vi "New Main.vi"() -> ()   [LabVIEW 2020]
panel:
  in  "Charging Voltage":dbl
  out "Total\nTemperature Change":dbl=nan
  out "Energy Loss":dbl=nan
  out "Power Loss":dbl=nan
  out "Charging Time":dbl=nan
  in  "Charing Current":dbl
  in  "Plot If Lit Up, Calculate Single if Not":bool=TRUE
  out "Results":cluster{"Output Array":dbl[], "Array y":dbl[]}(graph)
  in  "Upper Bound":dbl=2500.0
  in  "Number of Steps":dbl=2500.0
  in  "Lower Bound":dbl
  in  "Dependent Variable":u16(ring)=11 items=["Cap: Capacitance of 1 Pair NS", "Cap: Energy", "Cap: 1 NS Pair Energy / Mass", "Cap: 1 NS Pair Energy / Volume", "Cap: Impedance", "Cap: Power", "Cap: Chip Energy / Mass", "Cap: Chip Energy / Volume", "Cap: Chip Capacitance", "Cap: Chip Energy", "Cap: Chip Energy Wh", "Cap: Wh / kg", "Cap: Wh / m3", "Cap: Chip Impedance", "Cap: Chip Power", "Cap: Wh / Lit", "Cap: Energy Density Wh / m3", "Cap: J in 1 NS Pair with Gap", "Cap: Energy (Wh / m3) / 1 NS Pair with Gap", "Functionalization Molecule: Volume of Molecule", "Functionalization Molecule: Area of Molecule on CNT Surface", "Functionalization Molecule: Molecule Area with Gap", "Functionalization Molecule: Molecule Length", "Analyte Attached to Functionalized NS: Capacitance Functional Analyte per Unit Area", "Analyte Attached to Functionalized NS: Capacitance per CNT Analyte", "Analyte Attached to Functionalized NS: Capacitance Functional Analyte per NS", "Analyte Attached to Functionalized NS: Capacitance Functional Analyte per NS 2", "Analyte Molecule: Volume of Molecule Analyte", "Analyte Molecule: Area of Molecule on CNT Surface Analyte", "Analyte Molecule: Molecule Area with Gap Analyte", "Analyte Molecule: Molecule Length Analyte", "Molecule Functionalization: Number of Molecules on 1 CNT (Functionalized)", "Molecule Functionalization: Total Functionalized Molecules on NS", "Molecule Functionalization: Concentration on 1 NS (moles / m3)", "Molecule Functionalization: Concentration; M", "Capacitance of Functional Molecule on NS: Capacitance Functional Molecule per Unit Area", "Capacitance of Functional Molecule on NS: Capacitance per CNT (Functional)", "Capacitance of Functional Molecule on NS: Capacitance Functional Molecules per NS", "Capacitance of Functional Molecule on NS: Capacitance Functional Molecules per NS 2", "Constants: e0; Permitivity of Free Space", "Constants: c; Charge on e", "Constants: F; eN_A (Faraday's Constant)", "Constants: kB; Boltzmann Constant", "Constants: NA; Avagadro Number", "Constants: R=kN_A; Gas Constant", "EDL: C in M", "EDL: C_EDL / A", "EDL: d; EDL Length", "EDL: C EDL by d", "EDL: C EDL by d with cosh Factor", "EDL: C_EDL / 1 CNT", "EDL: C_EDL / 1 NS", "Potentiostat/Echem: Rf for Max I; R+C (EDL+Funct)", "Potentiostat/Echem: Rf for Max I; R+C (EDL+Funct+Analyte)", "Potentiostat/Echem: Capacitance of ELD & Functionalization", "Potentiostat/Echem: Impedance of EDL & Functionalization", "Potentiostat/Echem: Capacitance of ELD & Functionalization Analyte", "Potentiostat/Echem: Impedance of EDL & Functionalization Analyte", "Potentiostat/Echem: Total Impedance Rs +C (EDS+Funct)", "Potentiostat/Echem: Total Impedance Rs+C(EDS+Funct+Analyte)", "Potentiostat/Echem: Delta Total Impedance", "Potentiostat/Echem: Delta C", "Potentiostat/Echem: |Z| of R+C (EDL+Funct)", "Potentiostat/Echem: |Z| of R+C (EDL+Funct+Analyte)", "Potentiostat/Echem: V_Zeta", "Potentiostat/Echem: Max I; R+C (EDL+Funct)", "Potentiostat/Echem: Max I; R+C (EDL+Funct+Analyte)", "Potentiostat/Echem: Delta I", "Mass/Volume of Chip: Volume of a Chip", "Mass/Volume of Chip: Mass of a Chip", "Mass/Volume of NS Pair: Volume 1 NS", "Mass/Volume of NS Pair: Volume 2 NS", "Mass/Volume of NS Pair: Volume NS Pair with Gap", "Mass/Volume of NS Pair: Mass 1 NS", "Mass/Volume of NS Pair: Mass 2 NS", "Mass/Volume of NS Pair: Mass NS Pair with Gap", "Mass/Volume of NS Pair: Volume Gap", "Mass/Volume of NS Pair: Mass Gap", "Gap B/W NS Material: Silicon Thickness Gap", "Gap B/W NS Material: SiO2 Thickness Gap", "Gap B/W NS Material: Dielectric Thickness Gap", "Gap B/W NS Material: Volume Si Gap", "Gap B/W NS Material: Volume SiO2 Gap", "Gap B/W NS Material: Volume Dielectric Gap", "Gap B/W NS Material: Mass Si Gap", "Gap B/W NS Material: Mass SiO2 Gap", "Gap B/W NS Material: Mass Dielectric Gap", "Gap B/W NS Material: Delta Temp Change Si Gap", "Gap B/W NS Material: Delta Temp Change SiO2 Gap", "Gap B/W NS Material: Delta Temp Change Dielectric Gap", "NS Material Stack: CNT Thickness (CNT Length)", "NS Material Stack: Dielectric Thickness", "NS Material Stack: m-mm CNT", "NS Material Stack: m-mm Dielectric", "NS Material Stack: Silicon Thickness", "NS Material Stack: SiO2 Thickness", "NS Material Stack: SiO2 Thickness 2", "NS Material Stack: M1 Thickness", "NS Material Stack: Al2O3 Thickness", "NS Material Stack: Al Thickness", "NS Material Stack: Fe Thickness", "NS Material Stack: CNT Thickness", "NS Material Stack: Dielectric Thickness", "NS Material Stack: Volume Si", "NS Material Stack: Volume SiO2", "NS Material Stack: Volume SiO2 2", "NS Material Stack: Volume M1", "NS Material Stack: Volume Al2O3", "NS Material Stack: Volume Al", "NS Material Stack: Volume Fe", "NS Material Stack: Volume CNT", "NS Material Stack: Volume Dielectric", "NS Material Stack: Mass Si", "NS Material Stack: Mass SiO2", "NS Material Stack: Mass SiO2 2", "NS Material Stack: Mass M1", "NS Material Stack: Mass Al2O3", "NS Material Stack: Mass Al", "NS Material Stack: Mass Fe", "NS Material Stack: Mass CNTs", "NS Material Stack: Mass Dielectric", "NS Material Stack: Delta Temp Change Si", "NS Material Stack: Delta Temp Change SiO2", "NS Material Stack: Delta Temp Change SiO2 2", "NS Material Stack: Delta Temp Change M1", "NS Material Stack: Delta Temp Change Al2O3", "NS Material Stack: Delta Temp Change Al", "NS Material Stack: Delta Temp Change Fe", "NS Material Stack: Delta Temp Change CNT", "NS Material Stack: Delta Temp Change Dielectric", "Extraneous: Heat Generated (Energy) by Current in Metal Films", "Extraneous: um in 1 inch", "Extraneous: Microns", "Chip: Area B/W NS", "Chip: Gap B/W NS", "Chip: Number of NS Pairs on Chip", "NS: NS Width", "NS: NS Length", "NS: NS Base Area", "NS: Surface Area of 1 NS", "NS: Number of CNTs in 1 NS", "CNT NS: Length of CNTs", "CNT NS: CNT Radius", "CNT NS: CNT Base Area", "CNT NS: Surface Area of 1 CNT", "CNT NS: Area 1 CNT & Gap", "Material Stack Constants: Si Density", "Material Stack Constants: SiO2 Density", "Material Stack Constants: SiO2 2 Density", "Material Stack Constants: M1 Density", "Material Stack Constants: Al2O3 Density", "Material Stack Constants: Al Density", "Material Stack Constants: Fe Density", "Material Stack Constants: CNT Density", "Material Stack Constants: Dielectric Density", "Material Stack Constants: Si Specific Heat Capacity", "Material Stack Constants: SiO2 Specific Heat Capacity", "Material Stack Constants: SiO2 2 Specific Heat Capacity", "Material Stack Constants: M1 Specific Heat Capacity", "Material Stack Constants: Al2O3 Specific Heat Capacity", "Material Stack Constants: Al Specific Heat Capacity", "Material Stack Constants: Fe Specific Heat Capacity", "Material Stack Constants: CNT Specific Heat Capacity", "Material Stack Constants: Dielectric Specific Heat Capacity", "Charging/Discharging: Charging Time", "Charging/Discharging: Dissipated Power Loss", "Charging/Discharging: Total Energy Dissipated", "Charging/Discharging: Total Temperature Change"]
  in  "Independent Variable":u16(ring)=48 items=["CNT Ns: Radius of CNTs", "CNT Ns: Length of CNTs", "CNT Ns: Gap Between CNTs", "CNT Ns: m-mm r", "CNT Ns: m-mm l", "CNT Ns: m-mm gap", "Extraneous: Energy (Heat; I^2R)", "Extraneous: Inches", "NS Stack: Silicon Thickness", "Ns Stack: Silicon Dioxide Thickness", "Ns Stack: Silicon Dioxide Thickness 2", "Ns Stack: Metal 1 (Ti)", "Ns Stack: Alumina Thickness", "Ns Stack: Aluminum Thickness", "Ns Stack: Fe Thickness", "Ns Stack: m-mm Si", "Ns Stack: m-mm SiO2", "Ns Stack: m-mm SiO2 2", "Ns Stack: m-mm M1", "Ns Stack: m-mm Al2O3", "Ns Stack: m-mm Al", "Ns Stack: m-mm Fe", "Ns: Width of Base", "Ns: Length of Base", "Ns: m-mm WB", "Ns: m-mm NS Base", "Chip: Gap B/W Ns", "Chip: Width of Chip", "Chip: Length of Chip", "Chip: Gap n-m", "Chip: m-mm WChip", "Chip: m-mm LChip", "Functionalization Molecule: Radius of Molecule", "Functionalization Molecule: Length of Molecule", "Functionalization Molecule: Gap between Molecules", "Functionalization Molecule: Dielectric of Molecule", "Functionalization Molecule: m-mm r Molecule", "Functionalization Molecule: m-mm L molecule", "Functionalization Molecule: m-mm Gap Molecules", "Analyte Molecule: Radius of Molecule Analyte", "Analyte Molecule: Length of Molecule Analyte", "Analyte Molecule: Gap Between Molecules Analyte", "Analyte Molecule: Dielectric of Molecule 2 Analyte", "Analyte Molecule: m-mm r Molecule Analyte", "Analyte Molecule: m-mm l Molecule Analyte", "Analyte Molecule: m-mm Gap Molecules Analyte", "Cap: Energy Density WH/Lit", "Cap: Er 2", "Cap: Voltage", "Cap: Frequency 2", "Cap: Freq Hz K; M Hz", "Potentiostat/Echem: Max V Out", "Potentiostat/Echem: Series Resistance of Solution", "Potentiostat/Echem: Frequency", "Potentiostat/Echem: Freq Hz-MHz", "EDL: Co; milimolar (moles/m3)", "EDL: Z", "EDL: Er", "EDL: T", "EDL: V zeta", "EDL: Co nM-M", "EDL: V nV-m V-V", "Charging/Discharging: Constant Current", "Charging/Discharging: Constant Voltage"]
  out "J in 1 NS pair with gap":dbl
  out "Energy (wh/m3) / 1 NS pari with gap":dbl
  out "Energy Density  WH/m3":dbl
  in  "Energy Density  WH/Lit":dbl
  out "1 NS Pair Energy / Volume":dbl=81481754920.80457
  out "1 NS Pair Energy / mass":dbl=20280779.906268623
  out "Chip Energy Wh":dbl=8.077556418468985
  out "WH/Lit":dbl=22633.820811334605
  out "WH/m3":dbl=22633820.811334606
  out "WH/Kg":dbl=5633.549973963506
  out "Chip Energy / Volume":dbl=81481754920.80458
  out "Chip Energy /Mass":dbl=20280779.906268623
  out "Chip Impedance":dbl=inf
  out "Chip Capacitance":dbl=0.009305344994076273
  out "Chip Energy":dbl=29079.20310648835
  out "Chip Power":dbl
  in  "Freq Hz K; M Hz":dbl
  out "Power":dbl
  in  "Frequency 2":dbl
  out "Impedance":dbl=inf
  in  "Voltage":dbl=10.0
  out "Energy":dbl=17.172757740052173
  out "Capacitance of 1 Pair NS":dbl=5.495282476816696e-06
  in  "er 2":dbl=350.0
  out "Rf for Max i;  R+ C (EDL+Funct)":dbl=nan
  out "Rf for Max i;  R+ C (EDL+Funct+ Analyte)":dbl=nan
  in  "Max V_out":dbl
  out "Delta i":dbl=nan
  out "Max i;  R+ C (EDL+Funct+ Analyte)":dbl=nan format="%#_9e"
  out "Max i;  R+ C (EDL+Funct)":dbl=nan format="%#_9e"
  out "V_Zeta":dbl
  out "|Z| of R+ C (EDL+Funct+Analyte)":dbl=nan
  out "|Z| of R+ C (EDL+Funct)":dbl=nan
  out "Delta Total Impedance":dbl=nan
  out "Total Impedance Rs+C(EDS+Funct+Analyte)":dbl=nan
  out "Total Impedance Rs+C(EDS+Funct)":dbl=nan
  in  "Series Resistance of Solution":dbl
  in  "Freq Hz-MHz":dbl
  out "Impedance of EDL & Functionalization & Analyte":dbl=nan
  out "Impedance of EDL & Functionalization":dbl=nan
  in  "Frequency":dbl=1000.0
  out "Delta C":dbl=nan
  out "Capacitance of ELD & Functionalization & Analyte":dbl=nan
  out "Capacitance of ELD & Functionalization":dbl=nan
  out "C_EDL/ 1 NS":dbl=nan
  out "C_EDL/ 1 CNT":dbl=nan
  out "C EDL by d with Cosh Factor":dbl=nan format="%#_6e"
  out "C EDL by d":dbl=nan
  out "d; EDL Length":dbl=nan
  out "R=kN_a":dbl=8.314265387439999
  out "F=eN_a":dbl=5331991905204.0
  out "N_a; Avagadro no":dbl=6.022e+23
  in  "V  nV-m V-V":dbl
  out "C_EDL/ A":dbl=nan format="%#_6e"
  out "c; Charge on e":dbl=1.6021766208e-19
  in  "V zeta":dbl
  out "C in M":dbl
  in  "Co nM-M":dbl
  in  "T":dbl
  out "k; Boltzmann Constant":dbl=1.38064852e-23
  in  "Co; miliMolar (moles/m3)":dbl
  in  "er":dbl=1.0
  out "eo; Permitivity of Free Space":dbl=8.85418782e-12
  in  "z":dbl
  in  "Dielectric of Molecule 2 Analyte":dbl
  out "Capacitance Functinal Analyte  per unit area":dbl=nan
  out "Capaciatance per CNT Analyte":dbl=nan
  out "Capacitance Functional Analyte per NS":dbl=nan
  out "Capacitance Functional Analyte per NS 2":dbl=nan
  out "Capacitance Functional Molecules per NS 2":dbl=nan
  out "Capacitance Functional Molecules per NS":dbl=nan
  out "Capaciatance per CNT Functional":dbl=nan
  out "Capacitance Functinal Molecule  per unit area":dbl=nan
  in  "Dielectric of Molecule":dbl
  out "Concentration,  M":ext[unit]=inf
  out "Concentration on 1 NS (Moles/m3)":ext[unit]=inf
  out "Total Functionalized Molecules on NS":dbl=inf
  out "No of Molecules on 1 CNT Functionalized":dbl=inf
  out "Molecule Length Analyte":dbl
  out "Molecle Area with Gap Analyte":dbl
  out "Volume of Molecule Analyte":dbl
  out "Area of Molecule on CNT surface Analyte":dbl
  in  "m-nm Gap Molecules Analyte":dbl caption="m-nm Gap"
  in  "Gap Between Molecules Analyte":dbl caption="Gap Between CNTs"
  in  "m-nm l Molecule Analyte":dbl
  in  "m-nm r Molecule Analyte":dbl caption="m-nm r"
  in  "Length of Molecule Analyte":dbl caption="Length of CNTs"
  in  "Radius of Molecule Analyte":dbl caption="Radius of CNTs"
  out "Molecule Length":dbl
  out "Molecle Area with Gap":dbl
  out "Volume of Molecule":dbl
  out "Area of Molecule on CNT surface":dbl
  in  "m-nm Gap Molecules":dbl caption="m-nm Gap"
  in  "Gap Between Molecules":dbl caption="Gap Between CNTs"
  in  "m-nm l Molecule":dbl
  in  "m-nm r Molecule":dbl caption="m-nm r"
  in  "Length of Molecule":dbl caption="Length of CNTs"
  in  "Radius of Molecule":dbl caption="Radius of CNTs"
  out "Area B/W NS":dbl=1.2699999999999999e-07
  out "Length of CNTs  2":dbl=0.0005
  out "Gap B/w NS":dbl=4.9999999999999996e-06
  out "NS Width":dbl=4.9999999999999996e-06
  out "No of NS Pairs on Chip":dbl=1693.3333333333335
  in  "Gap n-m":dbl=-6.0
  in  "Gap B/W NS":dbl=5.0
  in  "m-nm LChip":dbl=-6.0
  in  "m-nm WChip":dbl=-6.0
  in  "Length of Chip":dbl=25400.0
  in  "Width of Chip":dbl=25400.0
  out "Surface Area 1 NS":dbl=0.008866316931494192
  out "# of CNTs in 1 NS":dbl=564444444.4444442 format="%#_6e"
  out "Area 1 CNT & Gap":dbl=2.2500000000000006e-16
  out "NS Length":dbl=0.0254
  out "NS Base Area":dbl=1.2699999999999999e-07
  out "CNT Radius":dbl=5e-09
  out "CNT Base Area":dbl=7.853981633974483e-17
  in  "m-nm NS Base":dbl=-6.0 caption="m-nm 4"
  in  "m-nm WB":dbl=-6.0
  in  "Length of Base":dbl=25400.0
  in  "Width of Base":dbl=5.0
  in  "m-nm Gap":dbl=-9.0
  in  "Gap Between CNTs":dbl=5.0
  out "Surface Area of 1 CNT":dbl=1.5708041807765307e-11
  in  "m-nm l":dbl=-6.0
  in  "m-nm r":dbl=-9.0
  in  "Length of CNTs":dbl=500.0
  in  "Radius of CNTs":dbl=5.0
  out "Mass of a Chip":dbl=0.0014338306140534668
  out "Volume of a Chip":dbl=3.568799314e-07
  out "Mass NS Pair with Gap":dbl=8.467503626299999e-07
  out "Volume NS Pair With Gap":dbl=2.10755865e-10
  out "Volume Gap":dbl=7.025195499999999e-11
  out "Mass Gap":dbl=6.327970770499999e-07
  out "Delta Temp Change \nDielectric Gap":dbl=nan
  out "Dielectric Thickness  \nGap":dbl=0.00050256
  out "Mass Dielectric \nGap":dbl=6.178271615999999e-07
  out "Volume Dielectric \nGap":dbl=6.382511999999999e-11
  out "Delta Temp Change\n SiO2 Gap":dbl=nan
  out "Mass SiO2 Gap":dbl=1.7441545e-10
  out "Sio2 Thickness Gap":dbl=6.05e-07
  out "Volume SiO2 Gap":dbl=7.6835e-14
  out "Volume Si Gap":dbl=6.3499999999999986e-12
  out "Silicon Thickness Gap":dbl=4.9999999999999996e-05
  out "Mass Si Gap":dbl=1.4795499999999997e-08
  out "Delta Temp Change\n Si Gap":dbl=nan
  out "Vol 2 NS":dbl=1.4050391e-10
  out "Mass 2 NS":dbl=2.1395328558e-07
  out "Mass 1 NS":dbl=1.0697664279e-07
  out "Volume 1 NS":dbl=7.0251955e-11
  out "um in 1 inch":dbl=25400.0
  out "Microns":dbl
  in  "Inches":dbl
  out "SiO2 Specfic Heat Capacity 2":dbl=730.0
  out "SilO2 Density 2":dbl=2270.0
  out "Dielectric Specfic Heat Capacity":dbl=120.0
  out "Dielectric Density":dbl=9680.0
  out "CNT Specfic Heat Capacity":dbl=500.0
  out "CNT Density":dbl=1400.0
  out "Fe Specfic Heat Capacity":dbl=462.0
  out "Fe Density":dbl=7874.0
  out "Al Specfic Heat Capacity":dbl=887.0
  out "Al Density":dbl=2710.0
  out "Al2O3 Specfic Heat Capacity":dbl=753.0
  out "Al2O3 Density":dbl=3965.0
  out "M1 Specfic Heat Capacity":dbl=540.0
  out "M1 Density":dbl=4520.0
  out "SiO2 Specfic Heat Capacity":dbl=730.0
  out "SilO2 Density":dbl=2270.0
  in  "Energy (Heat; I^2R)":dbl
  out "Heat Generated (Energy) by Current in Metal films":dbl=nan
  out "Silicon Specfic Heat Capacity":dbl=710.0
  out "Silicon Density":dbl=2330.0
  out "Delta Temp Change SiO2 2":dbl=nan
  out "Mass SiO2 2":dbl=8.6487e-11
  out "Volume SiO2 2":dbl=3.81e-14
  out "Delta Temp Change \nDielectric":dbl=nan
  out "Mass Dielectric":dbl=3.0733999999999997e-09
  out "Volume Dielectric":dbl=3.1749999999999996e-13
  out "Delta Temp Change CNT":dbl=nan
  out "Mass CNTs":dbl=8.89e-08
  out "Volume CNT":dbl=6.35e-11
  out "Delta Temp Change Fe":dbl=nan
  out "Mass Fe":dbl=4.9999899999999996e-12
  out "Volume Fe":dbl=6.35e-16
  out "Delta Temp Change Al":dbl=nan
  out "Mass  Al":dbl=1.7208499999999999e-12
  out "Volume Al":dbl=6.35e-16
  out "Delta Temp Change Al2O3":dbl=nan
  out "Mass Al2O3":dbl=2.5177749999999997e-11
  out "Volume Al2O3":dbl=6.3499999999999994e-15
  out "Delta Temp Change M1":dbl=nan
  out "Mass M1":dbl=2.8702e-12
  out "Volume M1":dbl=6.35e-16
  out "Delta Temp Change SiO2":dbl=nan
  out "Mass SiO2":dbl=8.6487e-11
  out "Volume SiO2":dbl=3.81e-14
  out "Dielectric Thickness  2":dbl=2.4999999999999998e-06
  out "CNT Thickness":dbl=0.0005
  out "Fe Thickness 2":dbl=5e-09
  out "Al Thickness":dbl=5e-09
  out "Al2O3 Thickness":dbl=5.0000000000000004e-08
  out "M1 Thickness":dbl=5e-09
  out "SiO2 Thickness 2":dbl=3.0000000000000004e-07
  out "Sio2 Thickness":dbl=3.0000000000000004e-07
  out "Silicon Thickness 2":dbl=4.9999999999999996e-05
  out "m-nm Dielectric":dbl=-6.0
  out "Dielectric Thickness":dbl=2.5
  out "m-nm CNT":dbl=-6.0
  out "CNT Thickness (CNT Length)":dbl=500.0
  in  "m-nm Fe":dbl=-9.0
  in  "Fe Thickness":dbl=5.0
  in  "m-nm Al":dbl=-9.0
  in  "Aluminum Thickness":dbl=5.0
  out "Delta Temp Change Si":dbl=nan
  out "Mass Si":dbl=1.4795499999999997e-08
  out "Volume Si":dbl=6.3499999999999986e-12
  in  "m-nm SiO2 2":dbl=-9.0
  in  "Silicon DiOxide Thickness  2":dbl=300.0
  in  "m-nm Al2O3":dbl=-9.0
  in  "m-nm M1":dbl=-9.0
  in  "Alumina Thickness":dbl=50.0
  in  "Metal 1 (Ti)":dbl=5.0
  in  "m-nm SiO2":dbl=-9.0
  in  "m-nm Si":dbl=-6.0
  in  "Silicon DiOxide Thickness":dbl=300.0
  in  "Silicon Thickness":dbl=50.0
  # "MAIN CONTROL"
  # "CNT Nanostructure"
  # "Nano Structure Material Stack"
  # "Constants for Materials in Stack"
  # "Charging/Discharging"
  # "CAP"
  # "Nano Structure"
  # "Chip CAP"
  # "Chip NanoStructure"
  # "CAP Design"
  # "Chip"
  # "Dielectric =1/2 of Gap B/w NS"
  # "TiO2: 4260 kg/m3\nHafnium Odide: 9680"
  # "GAP B/W NS  Material"
  # "Analyte Molecule"
  # "Functionalization Molecule"
  # "Analyte Attached to Functionalized  NanoStructure"
  # "Capacitance of Analyte Molecule on NanoStructure"
  # "Mass and Volume of NS Pair"
  # "Functionalized NanoStructure"
  # "Molecule Fnctionalization"
  # "Capacitance of Functional Molecule on NanoStructure"
  # "Mass and Volume of Chip"
  # "Echem & Electrical Signals"
  # "Electric Double Layer; EDL"
  # "Constants"
  # "Cosh(zeV_zeta/2kT)"
  # "Potentiostat"
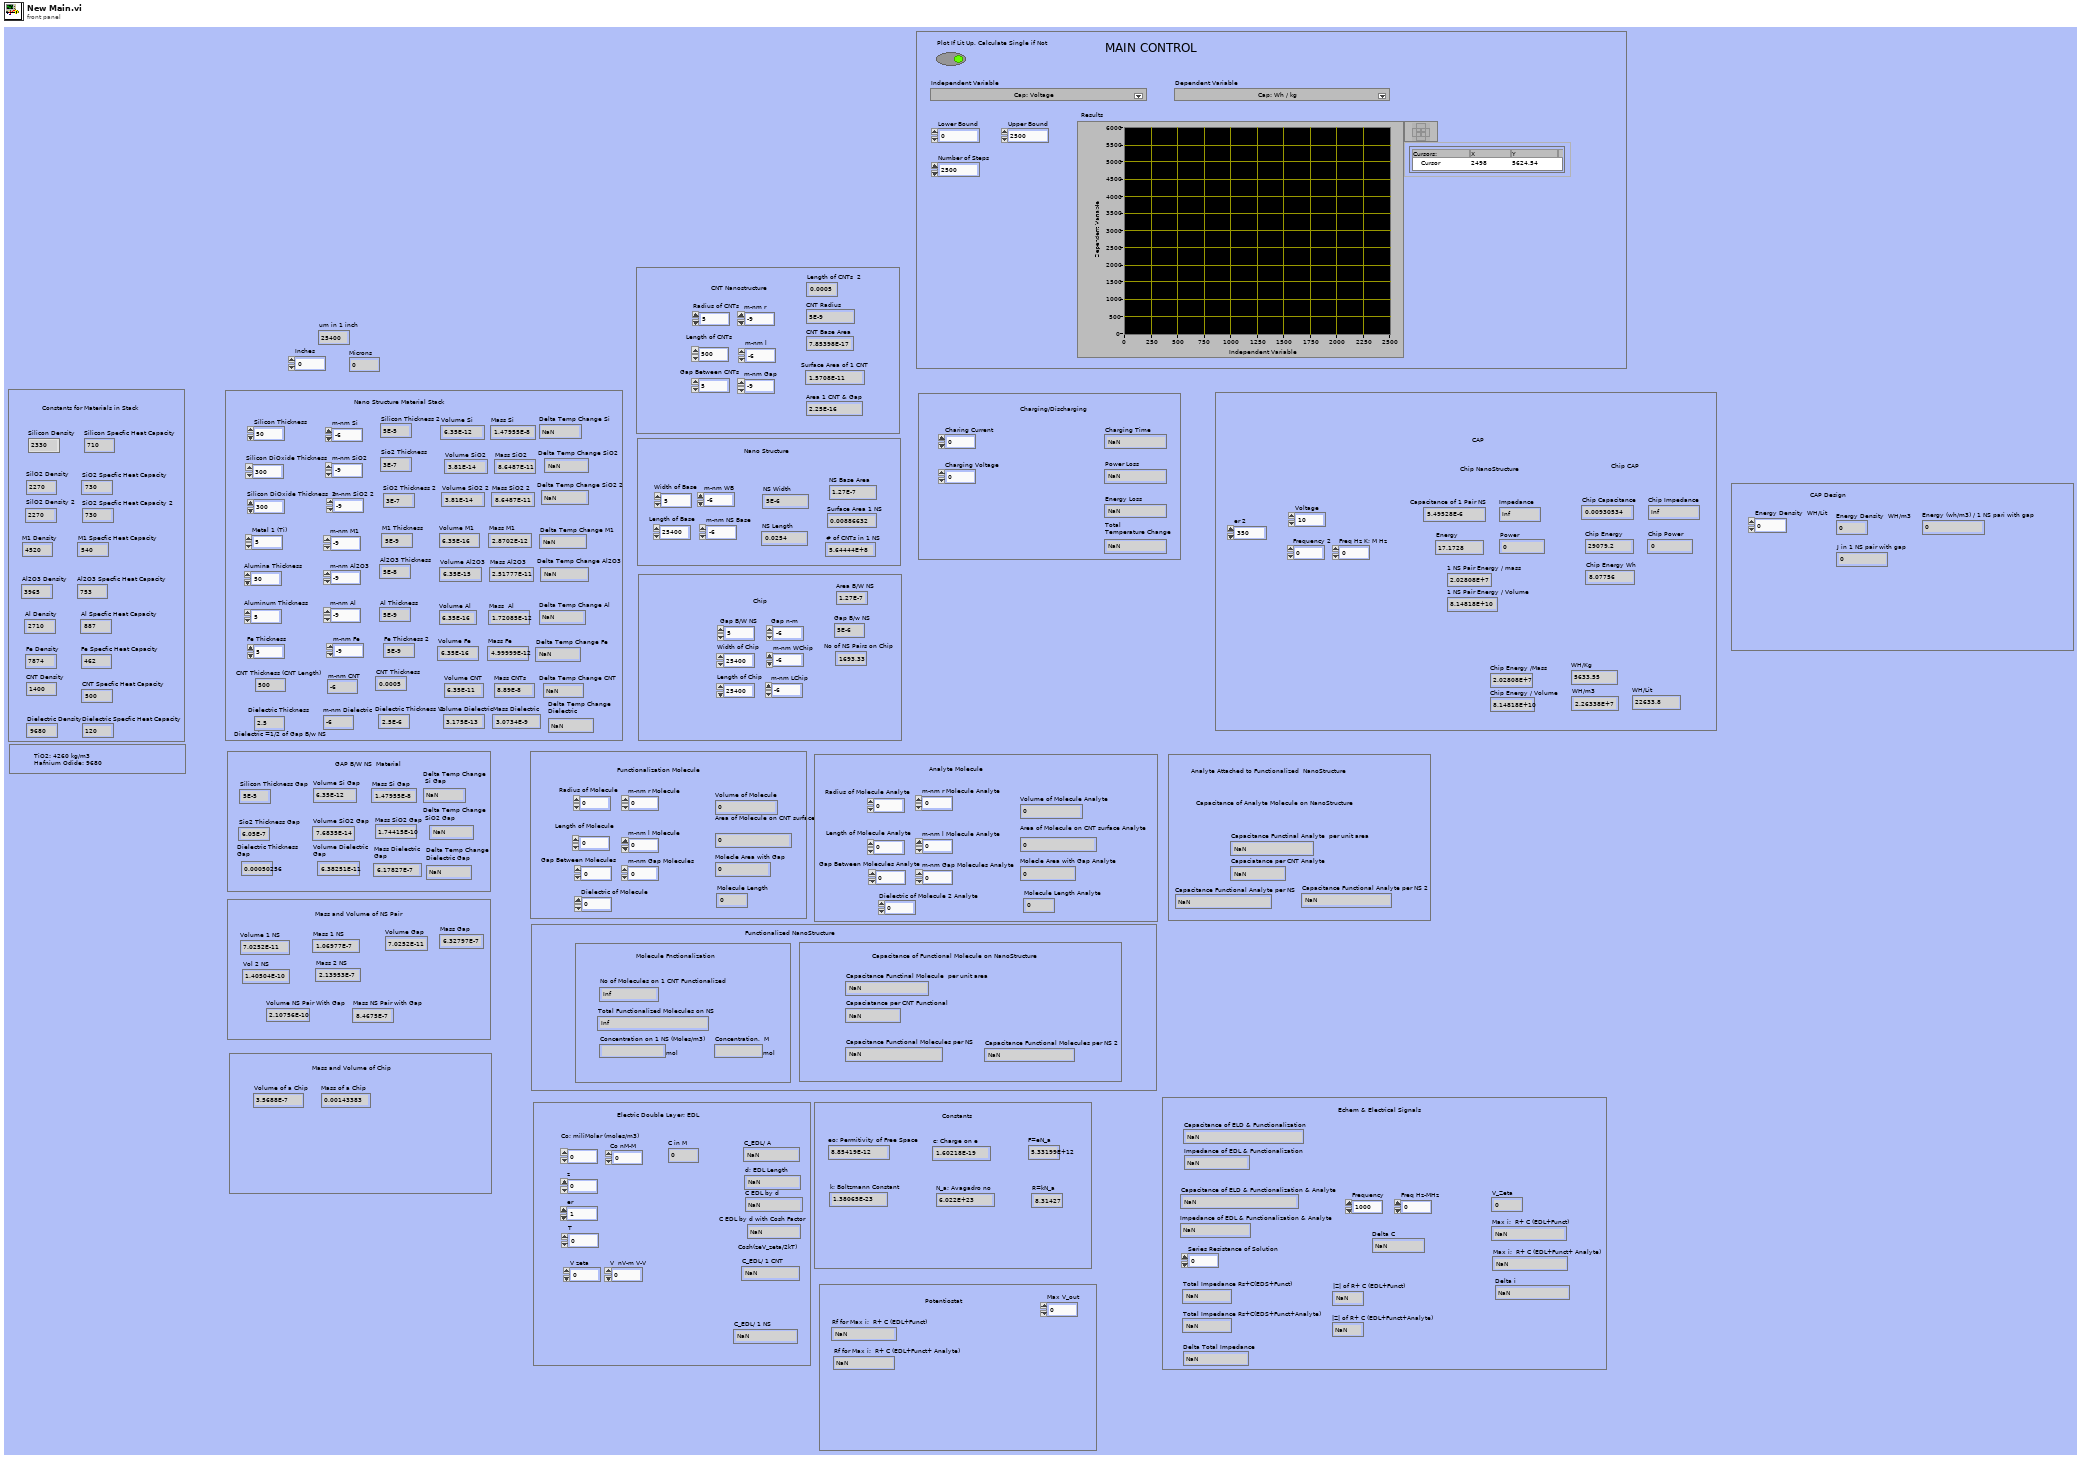
[diagram p1: front panel]
types:
  T1 = cluster{"Energy Density  WH/Lit":dbl, "er 2":dbl, "Voltage":dbl, "Frequency 2":dbl, "Freq Hz K; M Hz ":dbl}
  T2 = cluster{"Radius of CNTs":dbl, "Length of CNTs":dbl, "Gap Between CNTs ":dbl, "m-nm r":dbl, "m-nm l":dbl, "m-nm Gap":dbl}
  T3 = cluster{"Radius of Molecule Analyte":dbl, "Length of Molecule Analyte":dbl, "Gap Between Molecules Analyte":dbl, "Dielectric of Molecule 2 Analyte":dbl, "m-nm r Molecule Analyte":dbl, "m-nm l Molecule Analyte":dbl, "m-nm Gap Molecules Analyte":dbl}
  T4 = cluster{"Silicon Thickness":dbl, "Silicon DiOxide Thickness ":dbl, "Silicon DiOxide Thickness  2":dbl, "Metal 1 (Ti)":dbl, "Alumina Thickness  ":dbl, "Aluminum Thickness ":dbl, "Fe Thickness ":dbl, "m-nm Si":dbl, "m-nm SiO2":dbl, "m-nm SiO2 2":dbl, "m-nm M1":dbl, "m-nm Al2O3":dbl, "m-nm Al":dbl, "m-nm Fe":dbl}
  T5 = cluster{"Width of Base":dbl, "Length of Base":dbl, "m-nm WB":dbl, "m-nm NS Base":dbl}
  T6 = cluster{"Radius of Molecule":dbl, "Length of Molecule":dbl, "Gap Between Molecules":dbl, "Dielectric of Molecule":dbl, "m-nm r Molecule":dbl, "m-nm l Molecule":dbl, "m-nm Gap Molecules":dbl}
  T7 = cluster{"Gap B/W NS":dbl, "Width of Chip ":dbl, "Length of Chip":dbl, "Gap n-m":dbl, "m-nm WChip":dbl, "m-nm LChip ":dbl}
  T8 = cluster{"Co; miliMolar (moles/m3)":dbl, "z":dbl, "er":dbl, "T":dbl, "V zeta":dbl, "Co nM-M":dbl, "V  nV-m V-V":dbl}
  T9 = cluster{"Charing Current":dbl, "Charging Voltage":dbl}
  T10 = cluster{"Max V_out":dbl, "Series Resistance of Solution":dbl, "Frequency":dbl, "Freq Hz-MHz":dbl}
  T11 = cluster{"Radius of CNTs":dbl, "Length of CNTs":dbl, "Gap Between CNTs ":dbl, "m-nm r":dbl, "m-nm l":dbl, "m-nm Gap":dbl, "Energy (Heat; I^2R)":dbl, "Inches":dbl, "Silicon Thickness":dbl, "Silicon DiOxide Thickness ":dbl, "Silicon DiOxide Thickness  2":dbl, "Metal 1 (Ti)":dbl, "Alumina Thickness  ":dbl, "Aluminum Thickness ":dbl, "Fe Thickness ":dbl, "m-nm Si":dbl, "m-nm SiO2":dbl, "m-nm SiO2 2":dbl, "m-nm M1":dbl, "m-nm Al2O3":dbl, "m-nm Al":dbl, "m-nm Fe":dbl, "Width of Base":dbl, "Length of Base":dbl, "m-nm WB":dbl, "m-nm NS Base":dbl, "Gap B/W NS":dbl, "Width of Chip ":dbl, "Length of Chip":dbl, "Gap n-m":dbl, "m-nm WChip":dbl, "m-nm LChip ":dbl, "Radius of Molecule":dbl, "Length of Molecule":dbl, "Gap Between Molecules":dbl, "Dielectric of Molecule":dbl, "m-nm r Molecule":dbl, "m-nm l Molecule":dbl, "m-nm Gap Molecules":dbl, "Radius of Molecule Analyte":dbl, "Length of Molecule Analyte":dbl, "Gap Between Molecules Analyte":dbl, "Dielectric of Molecule 2 Analyte":dbl, "m-nm r Molecule Analyte":dbl, "m-nm l Molecule Analyte":dbl, "m-nm Gap Molecules Analyte":dbl, "Energy Density  WH/Lit":dbl, "er 2":dbl, "Voltage":dbl, "Frequency 2":dbl, "Freq Hz K; M Hz ":dbl, "Max V_out":dbl, "Series Resistance of Solution":dbl, "Frequency":dbl, "Freq Hz-MHz":dbl, "Co; miliMolar (moles/m3)":dbl, "z":dbl, "er":dbl, "T":dbl, "V zeta":dbl, "Co nM-M":dbl, "V  nV-m V-V":dbl, "Charing Current":dbl, "Charging Voltage":dbl}
  T12 = cluster{"Array Output Params[0]":dbl, "Array Output Params[1]":dbl, "Array Output Params[2]":dbl, "Array Output Params[3]":dbl, "Array Output Params[4]":dbl, "Array Output Params[5]":dbl, "Array Output Params[6]":dbl, "Array Output Params[7]":dbl, "Array Output Params[8]":dbl, "Array Output Params[9]":dbl, "Array Output Params[10]":dbl, "Array Output Params[11]":dbl, "Array Output Params[12]":dbl, "Array Output Params[13]":dbl, "Array Output Params[14]":dbl, "Array Output Params[15]":dbl, "Array Output Params[16]":dbl, "Array Output Params[17]":dbl, "Array Output Params[18]":dbl, "Array Output Params[19]":dbl, "Array Output Params[20]":dbl, "Array Output Params[21]":dbl, "Array Output Params[22]":dbl, "Array Output Params[23]":dbl, "Array Output Params[24]":dbl, "Array Output Params[25]":dbl, "Array Output Params[26]":dbl, "Array Output Params[27]":dbl, "Array Output Params[28]":dbl, "Array Output Params[29]":dbl, "Array Output Params[30]":dbl, "Array Output Params[31]":dbl, "Array Output Params[32]":dbl, "Array Output Params[33]":dbl, "Array Output Params[34]":dbl, "Array Output Params[35]":dbl, "Array Output Params[36]":dbl, "Array Output Params[37]":dbl, "Array Output Params[38]":dbl, "Array Output Params[39]":dbl, "Array Output Params[40]":dbl, "Array Output Params[41]":dbl, "Array Output Params[42]":dbl, "Array Output Params[43]":dbl, "Array Output Params[44]":dbl, "Array Output Params[45]":dbl, "Array Output Params[46]":dbl, "Array Output Params[47]":dbl, "Array Output Params[48]":dbl, "Array Output Params[49]":dbl, "Array Output Params[50]":dbl, "Array Output Params[51]":dbl, "Array Output Params[52]":dbl, "Array Output Params[53]":dbl, "Array Output Params[54]":dbl, "Array Output Params[55]":dbl, "Array Output Params[56]":dbl, "Array Output Params[57]":dbl, "Array Output Params[58]":dbl, "Array Output Params[59]":dbl, "Array Output Params[60]":dbl, "Array Output Params[61]":dbl, "Array Output Params[62]":dbl, "Array Output Params[63]":dbl, "Array Output Params[64]":dbl, "Array Output Params[65]":dbl, "Array Output Params[66]":dbl, "Array Output Params[67]":dbl, "Array Output Params[68]":dbl, "Array Output Params[69]":dbl, "Array Output Params[70]":dbl, "Array Output Params[71]":dbl, "Array Output Params[72]":dbl, "Array Output Params[73]":dbl, "Array Output Params[74]":dbl, "Array Output Params[75]":dbl, "Array Output Params[76]":dbl, "Array Output Params[77]":dbl, "Array Output Params[78]":dbl, "Array Output Params[79]":dbl, "Array Output Params[80]":dbl, "Array Output Params[81]":dbl, "Array Output Params[82]":dbl, "Array Output Params[83]":dbl, "Array Output Params[84]":dbl, "Array Output Params[85]":dbl, "Array Output Params[86]":dbl, "Array Output Params[87]":dbl, "Array Output Params[88]":dbl, "Array Output Params[89]":dbl, "Array Output Params[90]":dbl, "Array Output Params[91]":dbl, "Array Output Params[92]":dbl, "Array Output Params[93]":dbl, "Array Output Params[94]":dbl, "Array Output Params[95]":dbl, "Array Output Params[96]":dbl, "Array Output Params[97]":dbl, "Array Output Params[98]":dbl, "Array Output Params[99]":dbl, "Array Output Params[100]":dbl, "Array Output Params[101]":dbl, "Array Output Params[102]":dbl, "Array Output Params[103]":dbl, "Array Output Params[104]":dbl, "Array Output Params[105]":dbl, "Array Output Params[106]":dbl, "Array Output Params[107]":dbl, "Array Output Params[108]":dbl, "Array Output Params[109]":dbl, "Array Output Params[110]":dbl, "Array Output Params[111]":dbl, "Array Output Params[112]":dbl, "Array Output Params[113]":dbl, "Array Output Params[114]":dbl, "Array Output Params[115]":dbl, "Array Output Params[116]":dbl, "Array Output Params[117]":dbl, "Array Output Params[118]":dbl, "Array Output Params[119]":dbl, "Array Output Params[120]":dbl, "Array Output Params[121]":dbl, "Array Output Params[122]":dbl, "Array Output Params[123]":dbl, "Array Output Params[124]":dbl, "Array Output Params[125]":dbl, "Array Output Params[126]":dbl, "Array Output Params[127]":dbl, "Array Output Params[128]":dbl, "Array Output Params[129]":dbl, "Array Output Params[130]":dbl, "Array Output Params[131]":dbl, "Array Output Params[132]":dbl, "Array Output Params[133]":dbl, "Array Output Params[134]":dbl, "Array Output Params[135]":dbl, "Array Output Params[136]":dbl, "Array Output Params[137]":dbl, "Array Output Params[138]":dbl, "Array Output Params[139]":dbl, "Array Output Params[140]":dbl, "Array Output Params[141]":dbl, "Array Output Params[142]":dbl, "Array Output Params[143]":dbl, "Array Output Params[144]":dbl, "Array Output Params[145]":dbl, "Array Output Params[146]":dbl, "Array Output Params[147]":dbl, "Array Output Params[148]":dbl, "Array Output Params[149]":dbl, "Array Output Params[150]":dbl, "Array Output Params[151]":dbl, "Array Output Params[152]":dbl, "Array Output Params[153]":dbl, "Array Output Params[154]":dbl, "Array Output Params[155]":dbl, "Array Output Params[156]":dbl, "Array Output Params[157]":dbl, "Array Output Params[158]":dbl, "Array Output Params[159]":dbl, "Array Output Params[160]":dbl, "Array Output Params[161]":dbl, "Array Output Params[162]":dbl, "Array Output Params[163]":dbl, "Array Output Params[164]":dbl, "Array Output Params[165]":dbl, "Array Output Params[166]":dbl, "Array Output Params[167]":dbl}
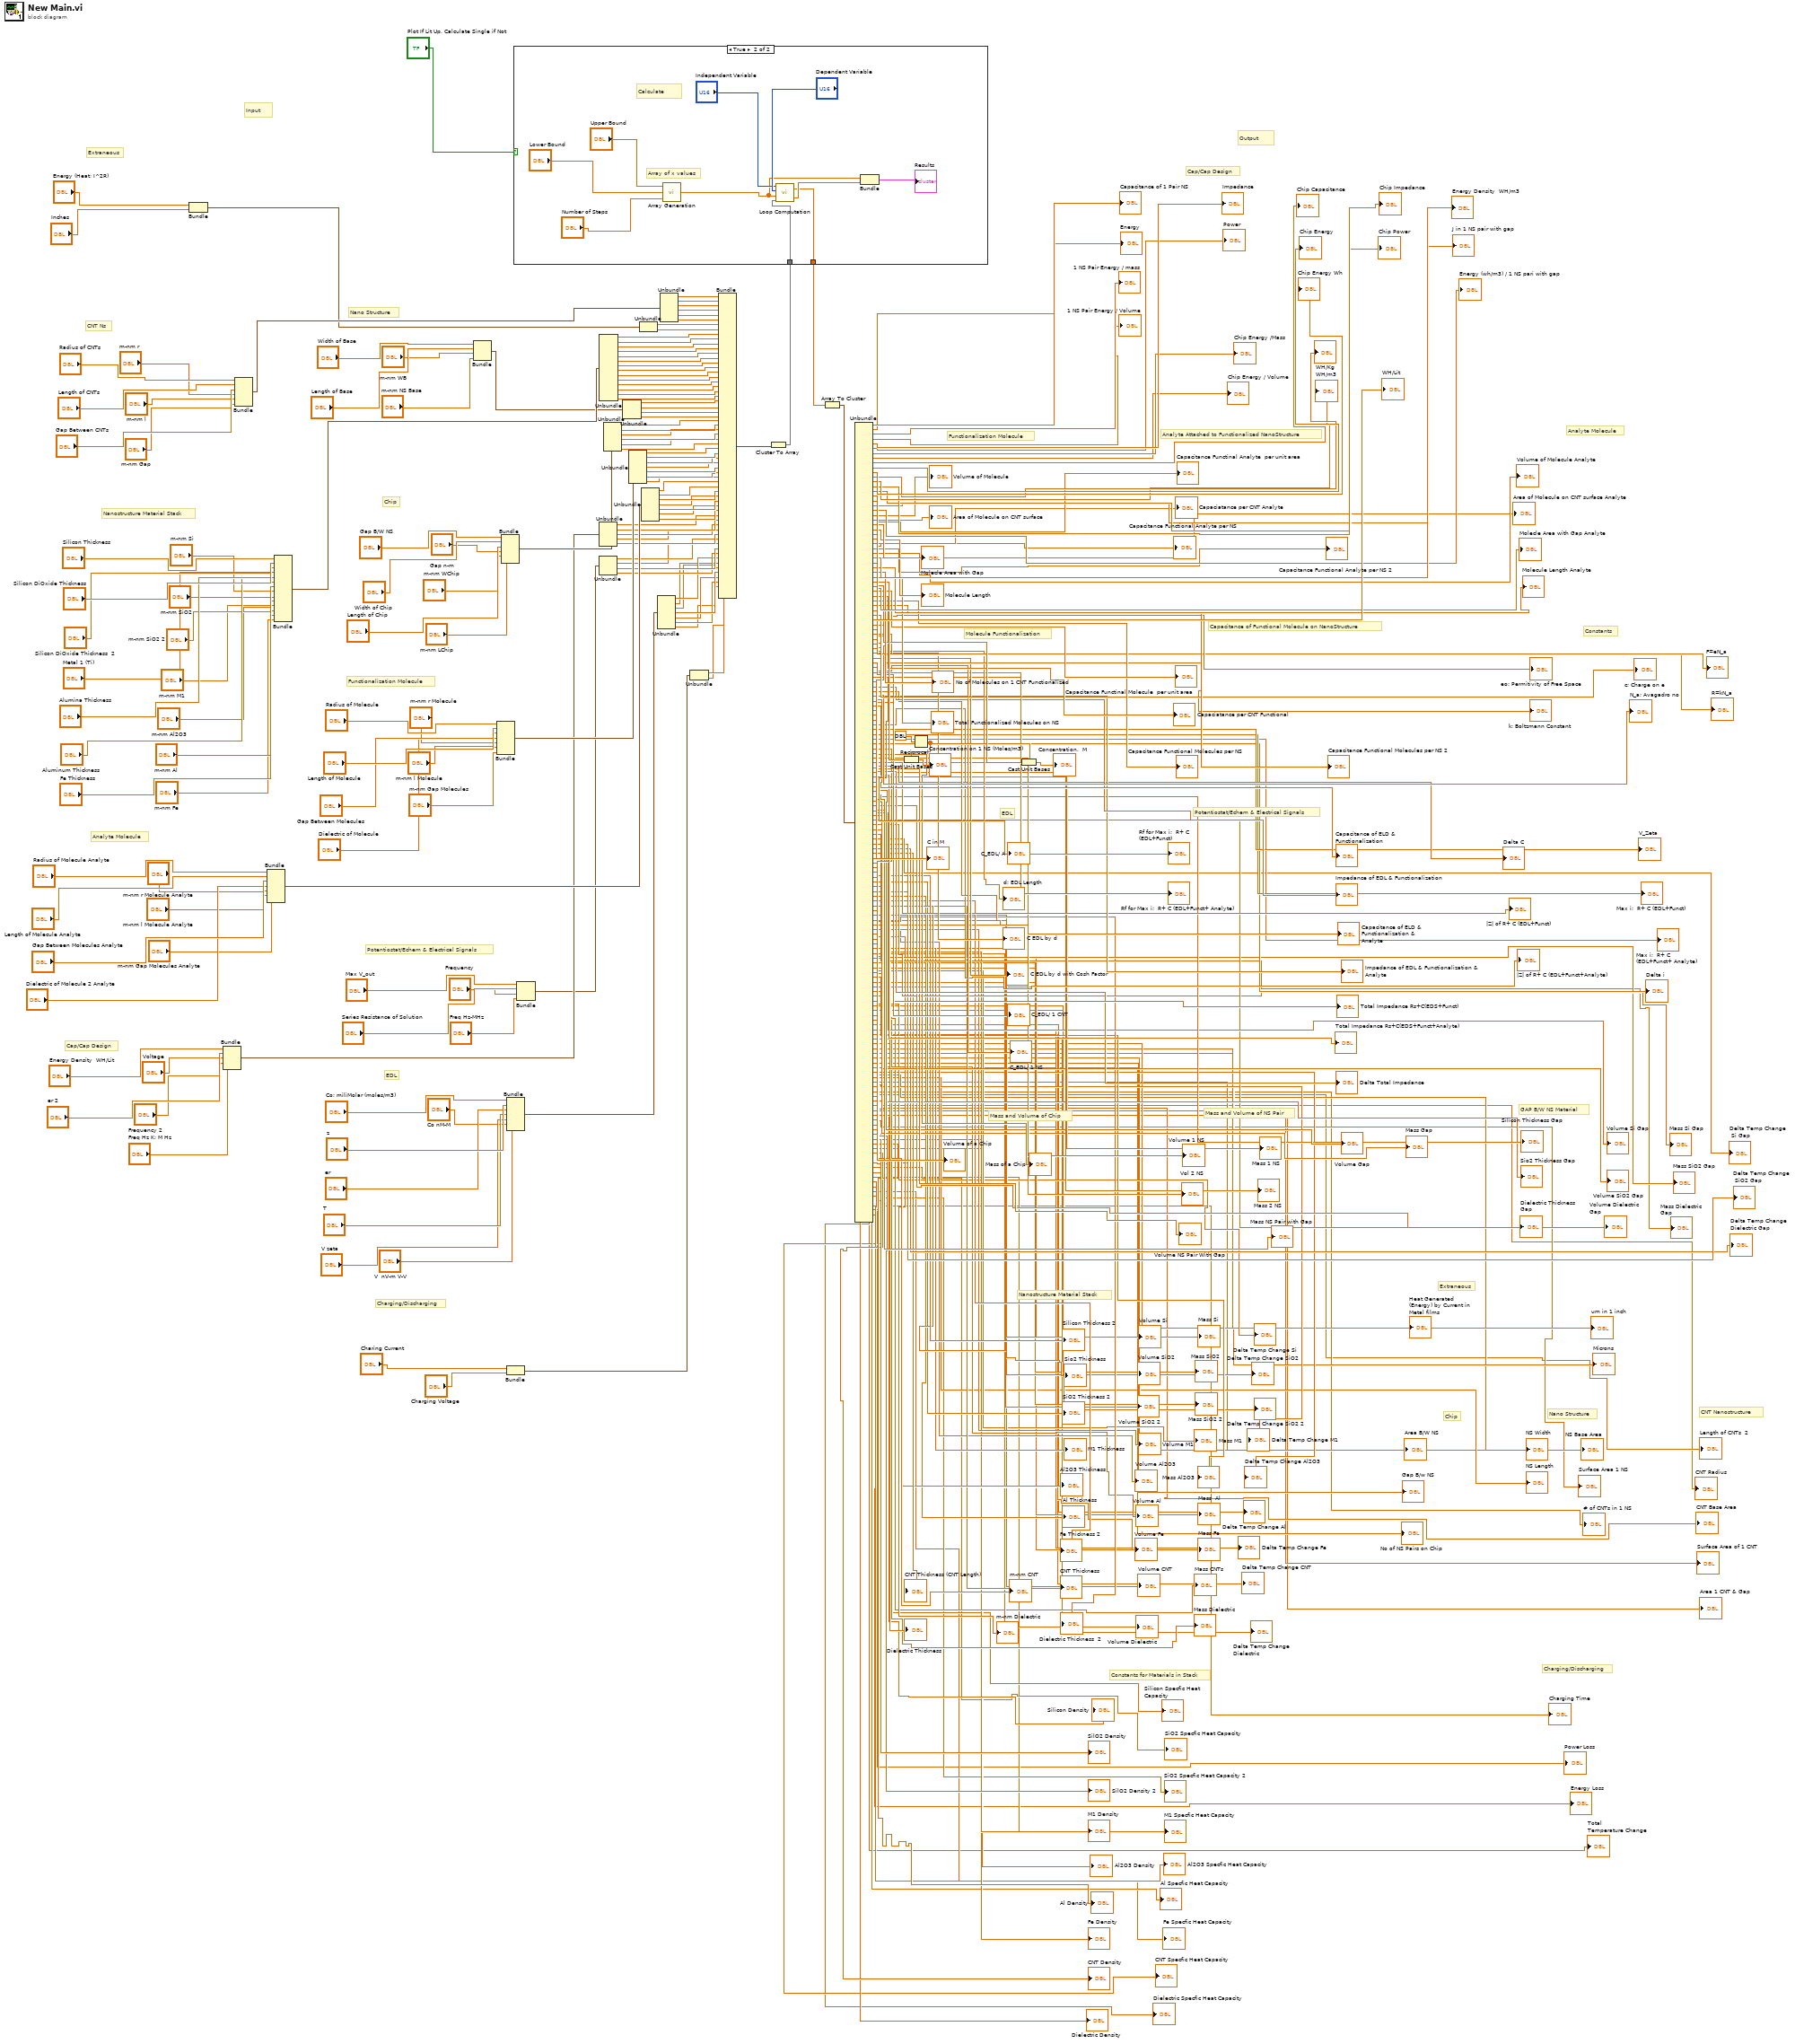
[diagram p0: block diagram]
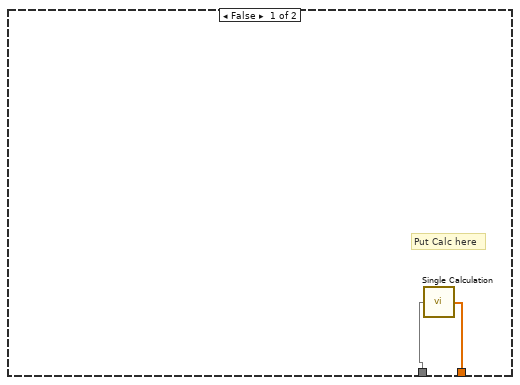
[diagram p2: hidden frame]
diagram:
  # "Charging/Discharging"
  # "Charging/Discharging"
  # "Input"
  # "Constants for Materials in Stack"
  # "CNT Nanostructure"
  # "Nano Structure"
  # "Chip"
  # "Extraneous"
  # "Nanostructure Material Stack"
  # "GAP B/W NS Material"
  # "Mass and Volume of NS Pair"
  # "Mass and Volume of Chip"
  # "Potentiostat/Echem & Electrical Signals"
  # "EDL"
  # "Constants"
  # "Capacitance of Functional Molecule on NanoStructure"
  # "Molecule Functionalization"
  # "Functionalization Molecule"
  # "Analyte Molecule"
  # "Analyte Attached to Functionalized NanoStructure"
  # "Cap/Cap Design"
  # "Output"
  # "EDL"
  # "Potentiostat/Echem & Electrical Signals"
  # "Cap/Cap Design"
  # "Analyte Molecule"
  # "Functionalization Molecule"
  # "Chip"
  # "Nano Structure"
  # "Nanostructure Material Stack"
  # "Extraneous"
  # "CNT Ns"
  n1 = Bundle("Energy (Heat; I^2R)"="Energy (Heat; I^2R)", "Inches"="Inches") -> (w247:cluster{"Energy (Heat; I^2R)":dbl, "Inches":dbl})  [unwired: 1 in]
  n2 = Bundle("Energy Density  WH/Lit"="Energy Density  WH/Lit", "er 2"="er 2", "Voltage"="Voltage", "Frequency 2"="Frequency 2", "Freq Hz K; M Hz"="Freq Hz K; M Hz") -> (w201:T1)  [unwired: 1 in]
  n3 = Bundle("Radius of CNTs"="Radius of CNTs", "Length of CNTs"="Length of CNTs", "Gap Between CNTs"="Gap Between CNTs", "m-nm r"="m-nm r", "m-nm l"="m-nm l", "m-nm Gap"="m-nm Gap") -> (w254:T2)  [unwired: 1 in]
  n4 = Bundle("Radius of Molecule Analyte"="Radius of Molecule Analyte", "Length of Molecule Analyte"="Length of Molecule Analyte", "Gap Between Molecules Analyte"="Gap Between Molecules Analyte", "Dielectric of Molecule 2 Analyte"="Dielectric of Molecule 2 Analyte", "m-nm r Molecule Analyte"="m-nm r Molecule Analyte", "m-nm l Molecule Analyte"="m-nm l Molecule Analyte", "m-nm Gap Molecules Analyte"="m-nm Gap Molecules Analyte") -> (w209:T3)  [unwired: 1 in]
  n5 = Bundle("Silicon Thickness"="Silicon Thickness", "Silicon DiOxide Thickness"="Silicon DiOxide Thickness", "Silicon DiOxide Thickness  2"="Silicon DiOxide Thickness  2", "Metal 1 (Ti)"="Metal 1 (Ti)", "Alumina Thickness"="Alumina Thickness", "Aluminum Thickness"="Aluminum Thickness", "Fe Thickness"="Fe Thickness", "m-nm Si"="m-nm Si", "m-nm SiO2"="m-nm SiO2", "m-nm SiO2 2"="m-nm SiO2 2", "m-nm M1"="m-nm M1", "m-nm Al2O3"="m-nm Al2O3", "m-nm Al"="m-nm Al", "m-nm Fe"="m-nm Fe") -> (w244:T4)  [unwired: 1 in]
  n6 = Bundle("Width of Base"="Width of Base", "Length of Base"="Length of Base", "m-nm WB"="m-nm WB", "m-nm NS Base"="m-nm NS Base") -> (w229:T5)  [unwired: 1 in]
  n7 = Bundle("Radius of Molecule"="Radius of Molecule", "Length of Molecule"="Length of Molecule", "Gap Between Molecules"="Gap Between Molecules", "Dielectric of Molecule"="Dielectric of Molecule", "m-nm r Molecule"="m-nm r Molecule", "m-nm l Molecule"="m-nm l Molecule", "m-nm Gap Molecules"="m-nm Gap Molecules") -> (w217:T6)  [unwired: 1 in]
  n8 = Bundle("Gap B/W NS"="Gap B/W NS", "Width of Chip"="Width of Chip", "Length of Chip"="Length of Chip", "Gap n-m"="Gap n-m", "m-nm WChip"="m-nm WChip", "m-nm LChip"="m-nm LChip") -> (w224:T7)  [unwired: 1 in]
  n9 = Bundle("Co; miliMolar (moles/m3)"="Co; miliMolar (moles/m3)", "z"="z", "er"="er", "T"="T", "V zeta"="V zeta", "Co nM-M"="Co nM-M", "V  nV-m V-V"="V  nV-m V-V") -> (w190:T8)  [unwired: 1 in]
  n10 = Bundle("Charing Current"="Charing Current", "Charging Voltage"="Charging Voltage") -> (w2:T9)  [unwired: 1 in]
  n11 = Bundle("Max V_out"="Max V_out", "Series Resistance of Solution"="Series Resistance of Solution", "Frequency"="Frequency", "Freq Hz-MHz"="Freq Hz-MHz") -> (w195:T10)  [unwired: 1 in]
  n12 = Unbundle(w201) -> ("Energy Density  WH/Lit"=w200:dbl, "er 2"=w199:dbl, "Voltage"=w198:dbl, "Frequency 2"=w197:dbl, "Freq Hz K; M Hz"=w196:dbl)
  n13 = Unbundle(w195) -> ("Max V_out"=w194:dbl, "Series Resistance of Solution"=w193:dbl, "Frequency"=w192:dbl, "Freq Hz-MHz"=w191:dbl)
  n14 = Unbundle(w244) -> ("Silicon Thickness"=w243:dbl, "Silicon DiOxide Thickness"=w242:dbl, "Silicon DiOxide Thickness  2"=w241:dbl, "Metal 1 (Ti)"=w240:dbl, "Alumina Thickness"=w239:dbl, "Aluminum Thickness"=w238:dbl, "Fe Thickness"=w237:dbl, "m-nm Si"=w236:dbl, "m-nm SiO2"=w235:dbl, "m-nm SiO2 2"=w234:dbl, "m-nm M1"=w233:dbl, "m-nm Al2O3"=w232:dbl, "m-nm Al"=w231:dbl, "m-nm Fe"=w230:dbl)
  n15 = Unbundle(w224) -> ("Gap B/W NS"=w223:dbl, "Width of Chip"=w222:dbl, "Length of Chip"=w221:dbl, "Gap n-m"=w220:dbl, "m-nm WChip"=w219:dbl, "m-nm LChip"=w218:dbl)
  n16 = Unbundle(w229) -> ("Width of Base"=w228:dbl, "Length of Base"=w227:dbl, "m-nm WB"=w226:dbl, "m-nm NS Base"=w225:dbl)
  n17 = Unbundle(w217) -> ("Radius of Molecule"=w216:dbl, "Length of Molecule"=w215:dbl, "Gap Between Molecules"=w214:dbl, "Dielectric of Molecule"=w213:dbl, "m-nm r Molecule"=w212:dbl, "m-nm l Molecule"=w211:dbl, "m-nm Gap Molecules"=w210:dbl)
  n18 = Unbundle(w247) -> ("Energy (Heat; I^2R)"=w246:dbl, "Inches"=w245:dbl)
  n19 = Unbundle(w209) -> ("Radius of Molecule Analyte"=w208:dbl, "Length of Molecule Analyte"=w207:dbl, "Gap Between Molecules Analyte"=w206:dbl, "Dielectric of Molecule 2 Analyte"=w205:dbl, "m-nm r Molecule Analyte"=w204:dbl, "m-nm l Molecule Analyte"=w203:dbl, "m-nm Gap Molecules Analyte"=w202:dbl)
  n20 = Unbundle(w190) -> ("Co; miliMolar (moles/m3)"=w189:dbl, "z"=w188:dbl, "er"=w187:dbl, "T"=w186:dbl, "V zeta"=w185:dbl, "Co nM-M"=w184:dbl, "V  nV-m V-V"=w183:dbl)
  n21 = Unbundle(w254) -> ("Radius of CNTs"=w253:dbl, "Length of CNTs"=w252:dbl, "Gap Between CNTs"=w251:dbl, "m-nm r"=w250:dbl, "m-nm l"=w249:dbl, "m-nm Gap"=w248:dbl)
  n22 = Unbundle(w2) -> ("Charing Current"=w4:dbl, "Charging Voltage"=w3:dbl)
  n23 = Bundle("Radius of CNTs"=w253, "Length of CNTs"=w252, "Gap Between CNTs"=w251, "m-nm r"=w250, "m-nm l"=w249, "m-nm Gap"=w248, "Energy (Heat; I^2R)"=w246, "Inches"=w245, "Silicon Thickness"=w243, "Silicon DiOxide Thickness"=w242, "Silicon DiOxide Thickness  2"=w241, "Metal 1 (Ti)"=w240, "Alumina Thickness"=w239, "Aluminum Thickness"=w238, "Fe Thickness"=w237, "m-nm Si"=w236, "m-nm SiO2"=w235, "m-nm SiO2 2"=w234, "m-nm M1"=w233, "m-nm Al2O3"=w232, "m-nm Al"=w231, "m-nm Fe"=w230, "Width of Base"=w228, "Length of Base"=w227, "m-nm WB"=w226, "m-nm NS Base"=w225, "Gap B/W NS"=w223, "Width of Chip"=w222, "Length of Chip"=w221, "Gap n-m"=w220, "m-nm WChip"=w219, "m-nm LChip"=w218, "Radius of Molecule"=w216, "Length of Molecule"=w215, "Gap Between Molecules"=w214, "Dielectric of Molecule"=w213, "m-nm r Molecule"=w212, "m-nm l Molecule"=w211, "m-nm Gap Molecules"=w210, "Radius of Molecule Analyte"=w208, "Length of Molecule Analyte"=w207, "Gap Between Molecules Analyte"=w206, "Dielectric of Molecule 2 Analyte"=w205, "m-nm r Molecule Analyte"=w204, "m-nm l Molecule Analyte"=w203, "m-nm Gap Molecules Analyte"=w202, "Energy Density  WH/Lit"=w200, "er 2"=w199, "Voltage"=w198, "Frequency 2"=w197, "Freq Hz K; M Hz"=w196, "Max V_out"=w194, "Series Resistance of Solution"=w193, "Frequency"=w192, "Freq Hz-MHz"=w191, "Co; miliMolar (moles/m3)"=w189, "z"=w188, "er"=w187, "T"=w186, "V zeta"=w185, "Co nM-M"=w184, "V  nV-m V-V"=w183, "Charing Current"=w4, "Charging Voltage"=w3) -> (w1:T11)  [unwired: 1 in]
  n24 = Cluster To Array(cluster=w1) -> (array=w182:dbl[])
  n25 = case shown="True" "Plot If Lit Up, Calculate Single if Not" {
    tunnel: w182 -> [w318 w325]
    tunnel: [w317 w319] -> w181
    frame False {
      # "Put Calc here"
      n26 = call "Single Calculation.vi"("Array Input"=w318) -> ("Array Output"=w317:dbl[])
    }
    frame True {
      # "Array of x values"
      # "Calculate"
      n27 = call "Array Generation.vi"("Number of Steps"="Number of Steps", "Lower Bound"="Lower Bound", "Upper Bound"="Upper Bound") -> ("Output Array"=w322:dbl[])
      n28 = call "Loop Computation.vi"("Array Params"=w325, "Array x"=w322, "y key"="Dependent Variable", "x key"="Independent Variable") -> ("Array y"=w321:dbl[], "Array Output Params"=w319:dbl[])
      n29 = Bundle("Output Array"=w322, "Array y"=w321) -> (→"Results":cluster{"Output Array":dbl[], "Array y":dbl[]})  [unwired: 1 in]
    }
  }
  n30 = Array To Cluster(array=w181) -> (cluster=w179:T12)
  n31 = Unbundle(w179) -> ("Array Output Params[0]"=→"Capacitance of 1 Pair NS":dbl, "Array Output Params[1]"=→"Energy":dbl, "Array Output Params[2]"=→"1 NS Pair Energy / mass":dbl, "Array Output Params[3]"=→"1 NS Pair Energy / Volume":dbl, "Array Output Params[4]"=→"Impedance":dbl, "Array Output Params[5]"=→"Power":dbl, "Array Output Params[6]"=→"Chip Energy /Mass":dbl, "Array Output Params[7]"=→"Chip Energy / Volume":dbl, "Array Output Params[8]"=→"Chip Capacitance":dbl, "Array Output Params[9]"=→"Chip Energy":dbl, "Array Output Params[10]"=→"Chip Energy Wh":dbl, "Array Output Params[11]"=→"WH/Kg":dbl, "Array Output Params[12]"=→"WH/m3":dbl, "Array Output Params[13]"=→"Chip Impedance":dbl, "Array Output Params[14]"=→"Chip Power":dbl, "Array Output Params[15]"=→"WH/Lit":dbl, "Array Output Params[16]"=→"Energy Density  WH/m3":dbl, "Array Output Params[17]"=→"J in 1 NS pair with gap":dbl, "Array Output Params[18]"=→"Energy (wh/m3) / 1 NS pari with gap":dbl, "Array Output Params[19]"=→"Volume of Molecule":dbl, "Array Output Params[20]"=→"Area of Molecule on CNT surface":dbl, "Array Output Params[21]"=→"Molecle Area with Gap":dbl, "Array Output Params[22]"=→"Molecule Length":dbl, "Array Output Params[23]"=→"Capacitance Functinal Analyte  per unit area":dbl, "Array Output Params[24]"=→"Capaciatance per CNT Analyte":dbl, "Array Output Params[25]"=→"Capacitance Functional Analyte per NS":dbl, "Array Output Params[26]"=→"Capacitance Functional Analyte per NS 2":dbl, "Array Output Params[27]"=→"Volume of Molecule Analyte":dbl, "Array Output Params[28]"=→"Area of Molecule on CNT surface Analyte":dbl, "Array Output Params[29]"=→"Molecle Area with Gap Analyte":dbl, "Array Output Params[30]"=→"Molecule Length Analyte":dbl, "Array Output Params[31]"=→"No of Molecules on 1 CNT Functionalized":dbl, "Array Output Params[32]"=→"Total Functionalized Molecules on NS":dbl, "Array Output Params[33]"=w145:dbl, "Array Output Params[34]"=w141:dbl, "Array Output Params[35]"=→"Capacitance Functinal Molecule  per unit area":dbl, "Array Output Params[36]"=→"Capaciatance per CNT Functional":dbl, "Array Output Params[37]"=→"Capacitance Functional Molecules per NS":dbl, "Array Output Params[38]"=→"Capacitance Functional Molecules per NS 2":dbl, "Array Output Params[39]"=→"eo; Permitivity of Free Space":dbl, "Array Output Params[40]"=→"c; Charge on e":dbl, "Array Output Params[41]"=→"F=eN_a":dbl, "Array Output Params[42]"=→"k; Boltzmann Constant":dbl, "Array Output Params[43]"=→"N_a; Avagadro no":dbl, "Array Output Params[44]"=→"R=kN_a":dbl, "Array Output Params[45]"=→"C in M":dbl, "Array Output Params[46]"=→"C_EDL/ A":dbl, "Array Output Params[47]"=→"d; EDL Length":dbl, "Array Output Params[48]"=→"C EDL by d":dbl, "Array Output Params[49]"=→"C EDL by d with Cosh Factor":dbl, "Array Output Params[50]"=→"C_EDL/ 1 CNT":dbl, "Array Output Params[51]"=→"C_EDL/ 1 NS":dbl, "Array Output Params[52]"=→"Rf for Max i;  R+ C (EDL+Funct)":dbl, "Array Output Params[53]"=→"Rf for Max i;  R+ C (EDL+Funct+ Analyte)":dbl, "Array Output Params[54]"=→"Capacitance of ELD & Functionalization":dbl, "Array Output Params[55]"=→"Impedance of EDL & Functionalization":dbl, "Array Output Params[56]"=→"Capacitance of ELD & Functionalization & Analyte":dbl, "Array Output Params[57]"=→"Impedance of EDL & Functionalization & Analyte":dbl, "Array Output Params[58]"=→"Total Impedance Rs+C(EDS+Funct)":dbl, "Array Output Params[59]"=→"Total Impedance Rs+C(EDS+Funct+Analyte)":dbl, "Array Output Params[60]"=→"Delta Total Impedance":dbl, "Array Output Params[61]"=→"Delta C":dbl, "Array Output Params[62]"=→"|Z| of R+ C (EDL+Funct)":dbl, "Array Output Params[63]"=→"|Z| of R+ C (EDL+Funct+Analyte)":dbl, "Array Output Params[64]"=→"V_Zeta":dbl, "Array Output Params[65]"=→"Max i;  R+ C (EDL+Funct)":dbl, "Array Output Params[66]"=→"Max i;  R+ C (EDL+Funct+ Analyte)":dbl, "Array Output Params[67]"=→"Delta i":dbl, "Array Output Params[68]"=→"Volume of a Chip":dbl, "Array Output Params[69]"=→"Mass of a Chip":dbl, "Array Output Params[70]"=→"Volume 1 NS":dbl, "Array Output Params[71]"=→"Vol 2 NS":dbl, "Array Output Params[72]"=→"Volume NS Pair With Gap":dbl, "Array Output Params[73]"=→"Mass 1 NS":dbl, "Array Output Params[74]"=→"Mass 2 NS":dbl, "Array Output Params[75]"=→"Mass NS Pair with Gap":dbl, "Array Output Params[76]"=→"Volume Gap":dbl, "Array Output Params[77]"=→"Mass Gap":dbl, "Array Output Params[78]"=→"Silicon Thickness Gap":dbl, "Array Output Params[79]"=→"Sio2 Thickness Gap":dbl, "Array Output Params[80]"=→"Dielectric Thickness  \nGap":dbl, "Array Output Params[81]"=→"Volume Si Gap":dbl, "Array Output Params[82]"=→"Volume SiO2 Gap":dbl, "Array Output Params[83]"=→"Volume Dielectric \nGap":dbl, "Array Output Params[84]"=→"Mass Si Gap":dbl, "Array Output Params[85]"=→"Mass SiO2 Gap":dbl, "Array Output Params[86]"=→"Mass Dielectric \nGap":dbl, "Array Output Params[87]"=→"Delta Temp Change\n Si Gap":dbl, "Array Output Params[88]"=→"Delta Temp Change\n SiO2 Gap":dbl, "Array Output Params[89]"=→"Delta Temp Change \nDielectric Gap":dbl, "Array Output Params[90]"=→"CNT Thickness (CNT Length)":dbl, "Array Output Params[91]"=→"Dielectric Thickness":dbl, "Array Output Params[92]"=→"m-nm CNT":dbl, "Array Output Params[93]"=→"m-nm Dielectric":dbl, "Array Output Params[94]"=→"Silicon Thickness 2":dbl, "Array Output Params[95]"=→"Sio2 Thickness":dbl, "Array Output Params[96]"=→"SiO2 Thickness 2":dbl, "Array Output Params[97]"=→"M1 Thickness":dbl, "Array Output Params[98]"=→"Al2O3 Thickness":dbl, "Array Output Params[99]"=→"Al Thickness":dbl, "Array Output Params[100]"=→"Fe Thickness 2":dbl, "Array Output Params[101]"=→"CNT Thickness":dbl, "Array Output Params[102]"=→"Dielectric Thickness  2":dbl, "Array Output Params[103]"=→"Volume Si":dbl, "Array Output Params[104]"=→"Volume SiO2":dbl, "Array Output Params[105]"=→"Volume SiO2 2":dbl, "Array Output Params[106]"=→"Volume M1":dbl, "Array Output Params[107]"=→"Volume Al2O3":dbl, "Array Output Params[108]"=→"Volume Al":dbl, "Array Output Params[109]"=→"Volume Fe":dbl, "Array Output Params[110]"=→"Volume CNT":dbl, "Array Output Params[111]"=→"Volume Dielectric":dbl, "Array Output Params[112]"=→"Mass Si":dbl, "Array Output Params[113]"=→"Mass SiO2":dbl, "Array Output Params[114]"=→"Mass SiO2 2":dbl, "Array Output Params[115]"=→"Mass M1":dbl, "Array Output Params[116]"=→"Mass Al2O3":dbl, "Array Output Params[117]"=→"Mass  Al":dbl, "Array Output Params[118]"=→"Mass Fe":dbl, "Array Output Params[119]"=→"Mass CNTs":dbl, "Array Output Params[120]"=→"Mass Dielectric":dbl, "Array Output Params[121]"=→"Delta Temp Change Si":dbl, "Array Output Params[122]"=→"Delta Temp Change SiO2":dbl, "Array Output Params[123]"=→"Delta Temp Change SiO2 2":dbl, "Array Output Params[124]"=→"Delta Temp Change M1":dbl, "Array Output Params[125]"=→"Delta Temp Change Al2O3":dbl, "Array Output Params[126]"=→"Delta Temp Change Al":dbl, "Array Output Params[127]"=→"Delta Temp Change Fe":dbl, "Array Output Params[128]"=→"Delta Temp Change CNT":dbl, "Array Output Params[129]"=→"Delta Temp Change \nDielectric":dbl, "Array Output Params[130]"=→"Heat Generated (Energy) by Current in Metal films":dbl, "Array Output Params[131]"=→"um in 1 inch":dbl, "Array Output Params[132]"=→"Microns":dbl, "Array Output Params[133]"=→"Area B/W NS":dbl, "Array Output Params[134]"=→"Gap B/w NS":dbl, "Array Output Params[135]"=→"No of NS Pairs on Chip":dbl, "Array Output Params[136]"=→"NS Width":dbl, "Array Output Params[137]"=→"NS Length":dbl, "Array Output Params[138]"=→"NS Base Area":dbl, "Array Output Params[139]"=→"Surface Area 1 NS":dbl, "Array Output Params[140]"=→"# of CNTs in 1 NS":dbl, "Array Output Params[141]"=→"Length of CNTs  2":dbl, "Array Output Params[142]"=→"CNT Radius":dbl, "Array Output Params[143]"=→"CNT Base Area":dbl, "Array Output Params[144]"=→"Surface Area of 1 CNT":dbl, "Array Output Params[145]"=→"Area 1 CNT & Gap":dbl, "Array Output Params[146]"=→"Silicon Density":dbl, "Array Output Params[147]"=→"SilO2 Density":dbl, "Array Output Params[148]"=→"SilO2 Density 2":dbl, "Array Output Params[149]"=→"M1 Density":dbl, "Array Output Params[150]"=→"Al2O3 Density":dbl, "Array Output Params[151]"=→"Al Density":dbl, "Array Output Params[152]"=→"Fe Density":dbl, "Array Output Params[153]"=→"CNT Density":dbl, "Array Output Params[154]"=→"Dielectric Density":dbl, "Array Output Params[155]"=→"Silicon Specfic Heat Capacity":dbl, "Array Output Params[156]"=→"SiO2 Specfic Heat Capacity":dbl, "Array Output Params[157]"=→"SiO2 Specfic Heat Capacity 2":dbl, "Array Output Params[158]"=→"M1 Specfic Heat Capacity":dbl, "Array Output Params[159]"=→"Al2O3 Specfic Heat Capacity":dbl, "Array Output Params[160]"=→"Al Specfic Heat Capacity":dbl, "Array Output Params[161]"=→"Fe Specfic Heat Capacity":dbl, "Array Output Params[162]"=→"CNT Specfic Heat Capacity":dbl, "Array Output Params[163]"=→"Dielectric Specfic Heat Capacity":dbl, "Array Output Params[164]"=→"Charging Time":dbl, "Array Output Params[165]"=→"Power Loss":dbl, "Array Output Params[166]"=→"Energy Loss":dbl, "Array Output Params[167]"=→"Total\nTemperature Change":dbl)
  n32 = Reciprocal(x=ext[unit] 6.0221408569999999998e+23) -> (1/x=w140:ext[unit])
  n33 = Cast Unit Bases(0:w145, 1:w140) -> (2:→"Concentration on 1 NS (Moles/m3)":dbl[unit])
  n34 = Cast Unit Bases(0:w141, 1:w140) -> (2:→"Concentration,  M":dbl[unit])
